vi "Read PLC Type.vi"(8 "error in (no error)":errorcluster, 10 "Symbol Name":string, 11 "TwinCAT ADS in":refnum<class "TwinCAT ADS.lvclass">) -> (0 "error out":errorcluster, 2 "PLC Type":T1, 3 "TwinCAT ADS out":refnum<class "TwinCAT ADS.lvclass">)   [LabVIEW 2018, in "TwinCAT ADS.lvclass"]
uses:
  TwinCAT ADS.lvclass
  Controls/PLC Type.ctl
  TwinCAT ADS.lvclass/TwinCAT ADS.ctl
  TwinCAT.Ads
  Get From Symbol Map.vi
  Get From Symbol Map Daemon.vi
  Get Symbol Map.vi
  Format String.vi
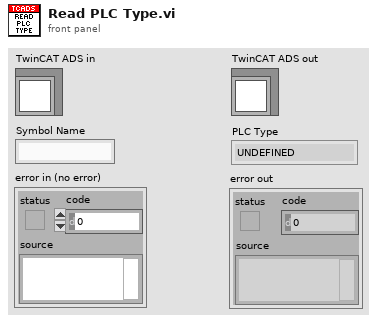
[diagram p1: front panel]
types:
  T1 = typedef "TwinCAT ADS.lvclass/PLC Type.ctl" = enum16{"UNDEFINED", "INT", "DINT", "REAL", "LREAL", "SINT", "BYTE", "UINT", "UDINT", "LINT", "ULINT", "STRING", "WSTRING", "BOOL", "TIME", "LTIME", "DATE", "DT", "TOD", "ARRAY", "JAGGED ARRAY", "STRUCT", "FUNCTION BLOCK", "UNION", "POINTER", "USER DEFINED"}
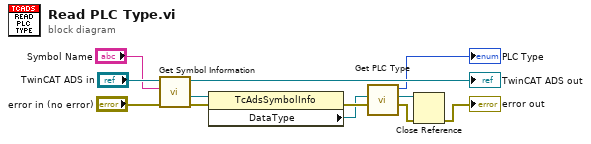
[diagram p0: block diagram]
diagram:
  n1 = call "Get Symbol Information.vi"("error in (no error)"="error in (no error)", "Symbol Name"="Symbol Name", "TwinCAT ADS in"="TwinCAT ADS in") -> ("error out"=w11:errorcluster, ".NET Symbol Information"=w10:refnum<k24>, "TwinCAT ADS out"=→"TwinCAT ADS out":refnum<class "TwinCAT ADS.lvclass">)  [unwired: 6 in]
  n2 = property class="TcAdsSymbolInfo"(reference=w10, error in=w11) -> (error out=w12:errorcluster, "DataType"=w9:refnum<k24>)  [unwired: 1 out]
  n3 = call "Get PLC Type.vi"("error in (no error)"=w12, ".NET AdsDataType in"=w9) -> ("error out"=w4:errorcluster, ".NET AdsDataType"=w5:refnum<k24>, "PLC Type"=→"PLC Type":T1)  [unwired: 7 in]
  n4 = Close Reference(reference=w5, error in (no error)=w4) -> (error out=→"error out":errorcluster)
